vi "Set Items.vi"(0 "Display State In":T1={"Prompt"="Click to add", "Listbox"=refnum, "Required"={"Strings"=[], "Bottom"=FALSE, "Italic"=FALSE, "FG"=0, "BG"=16777215, "Bold"=FALSE}, "Items"=[], "Req'd"=[], "Events"={"Items Changed"=refnum, "List Changed"=refnum}, "Max Rows"=-1, "Default name"=""}, 5 "Items":string[](array[string]), 7 "Required":string[](array[string]), 9 "Container State":T4, 11 "error in (no error)":errorcluster) -> (4 "Display State Out":T1={"Prompt"="Click to add", "Listbox"=refnum, "Required"={"Strings"=[], "Bottom"=FALSE, "Italic"=FALSE, "FG"=0, "BG"=16777215, "Bold"=FALSE}, "Items"=[], "Req'd"=[], "Events"={"Items Changed"=refnum, "List Changed"=refnum}, "Max Rows"=-1, "Default name"=""}, 8 "Merged Items":string[](array[string]), 10 "Nonrequired":string[](array[string]), 15 "error out":errorcluster)   [LabVIEW 2015, in "KListboxEx.xctl"]
uses:
  KListboxEx.xctl
  <vilib>/_xctls/Container State.ctl
  State.ctl
  Required.ctl
  Events.ctl
  Event Action.ctl
  <vilib>/_xctls/XControlSupport.lvlib
panel:
  # "Add Controls & Indicators that form the parameters of the method here. Hook them to the connector pane. Do not delete the controls & indicators that are already hooked to the connector pane.\n \nTo setup the parameters  for this method, right click on this item in the Project Tree & select \"Configure Method...\"."
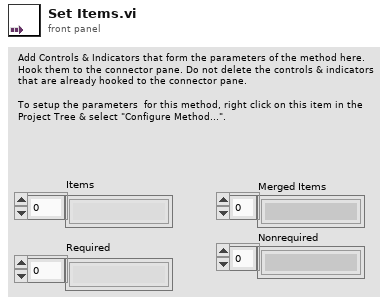
[diagram p1: front panel]
types:
  T1 = typedef "KListboxEx.xctl/State.ctl" = cluster{"Prompt":string, "Listbox":refnum<vi>, "Required":T2, "Items":string[], "Req'd":bool[], "Events":T3, "Max Rows":i32, "Default name":string}
  T2 = typedef "KListboxEx.xctl/Required.ctl" = cluster{"Strings":string[], "Bottom":bool, "Italic":bool, "FG":u32, "BG":u32, "Bold":bool}
  T3 = typedef "KListboxEx.xctl/Events.ctl" = cluster{"Items Changed":refnum<user-event>, "List Changed":refnum<user-event>}
  T4 = typedef "XControlSupport.lvlib/Container State.ctl" = cluster{"Indicator?":bool, "Run Mode?":bool, " Refnum":refnum<vi>}
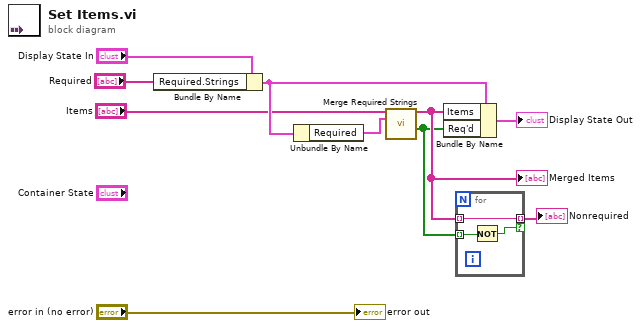
[diagram p0: block diagram]
diagram:
  n1 = Bundle By Name(cluster="Display State In", "Required.Strings"="Required") -> (w7:T1)
  n2 = Unbundle By Name(w7) -> ("Required"=w8:T2)
  n3 = call "Merge Required Strings.vi"("Strings In"="Items", "Required"=w8) -> ("Strings Out"=w4:string[], "Req'd"=w1:bool[])  [unwired: 12 in]
  "Merged Items" <- w4
  n4 = Bundle By Name(cluster=w7, "Items"=w4, "Req'd"=w1) -> (→"Display State Out":T1)
  n5 = for {
    tunnel: w4 -> [w13] mode=indexing
    tunnel: [w13] -> w2 mode=indexing if=w11
    tunnel: w1 -> [w12] mode=indexing
    n6 = Not(x=w12) -> (.not. x?=w11:bool)
  }
  "Nonrequired" <- w2
  "error out" <- "error in (no error)"
